vi "Configure Frequency Offset.vi"(8 "error in (no error)":errorcluster, 10 "Frequency Offset (0 Hz)":dbl, 11 "VISA resource name":refnum<visa-resource-name>) -> (0 "error out":errorcluster, 3 "VISA resource name out":refnum<visa-resource-name>)   [LabVIEW 2014, in "Agilent ESA PSA Series.lvlib"]
doc: "Configures the frequency offset of the spectrum analyzer"
uses:
  Agilent ESA PSA Series.lvlib
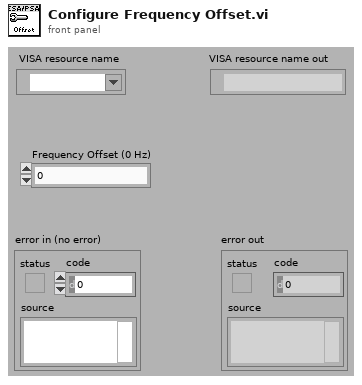
[diagram p1: front panel]
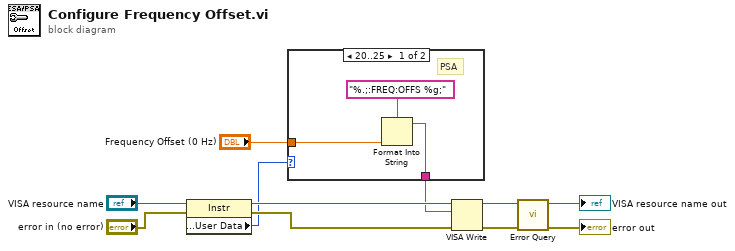
[diagram p0: block diagram]
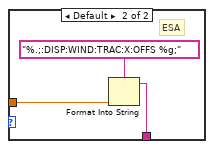
[diagram p2: hidden frame]
diagram:
  n1 = property on="Property Node" class="Instr"(reference="VISA resource name", error in="error in (no error)") -> (reference out=w4:refnum<visa-resource-name>, error out=w5:errorcluster, "General Settings:User Data"=w3:u32)
  n2 = case shown="20..25" w3 {
    tunnel: "Frequency Offset (0 Hz)" -> [w14 w16]
    tunnel: [w12 w15] -> w1
    frame 20..25 {
      # "PSA"
      n3 = Format Into String(format string="%.;:FREQ:OFFS %g;", w14) -> (resulting string=w12:string)  [unwired: 2 in, 1 out]
    }
    frame Default {
      # "ESA"
      n4 = Format Into String(format string="%.;:DISP:WIND:TRAC:X:OFFS %g;", w16) -> (resulting string=w15:string)  [unwired: 2 in, 1 out]
    }
  }
  n5 = VISA Write(VISA resource name=w4, write buffer=w1, error in (no error)=w5) -> (VISA resource name out=w11:refnum<visa-resource-name>, error out=w9:errorcluster)  [unwired: 1 out]
  n6 = call "Error Query.vi"("error in (no error)"=w9, "VISA resource name"=w11) -> ("error out"=→"error out":errorcluster, "VISA resource name out"=→"VISA resource name out":refnum<visa-resource-name>)  [unwired: 6 in, 2 out]
